vi "Stop Event Handler.vi"(8 "error in (no error)":errorcluster, 11 "EventHandler":refnum<class "IEventHandler.lvclass">) -> ()   [LabVIEW 2015, in "ActorEvents.lvlib" / "IEventHandler.lvclass"]
uses:
  IEventHandler.lvclass
  IEventHandler.lvclass/IEventHandler.ctl
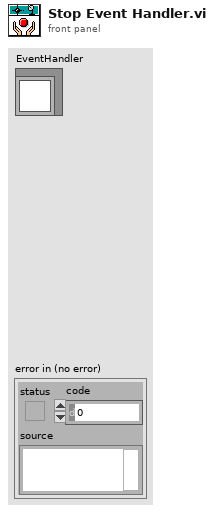
[diagram p1: front panel]
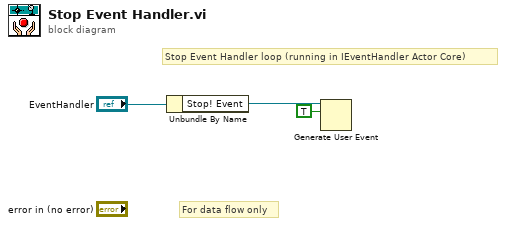
[diagram p0: block diagram]
diagram:
  # "For data flow only"
  # "Stop Event Handler loop (running in IEventHandler Actor Core)"
  n1 = Unbundle By Name("EventHandler") -> ("Stop! Event"=w2:refnum<user-event>)
  n2 = Generate User Event(user event=w2, event data cluster=TRUE ("event data")) -> ()  [unwired: 2 in, 2 out]
